vi "Read Scrubber.vi"(8 "error in":errorcluster, 11 "Options in":refnum<class "Options.lvclass">) -> (0 "error out":errorcluster, 2 "Scrubber":refnum<class "Scrubber.lvclass">, 3 "Options out":refnum<class "Options.lvclass">)   [LabVIEW 2020, in "Approval Tests.lvlib" / "Options.lvclass"]
uses:
  Options.lvclass
  Scrubber/Scrubber.lvclass
  Options.lvclass/Options.ctl
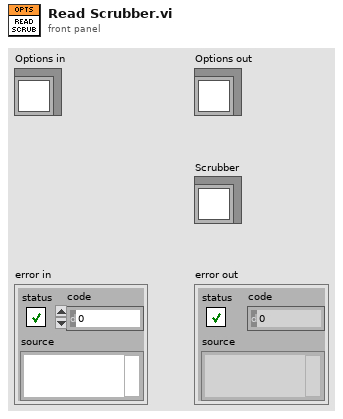
[diagram p1: front panel]
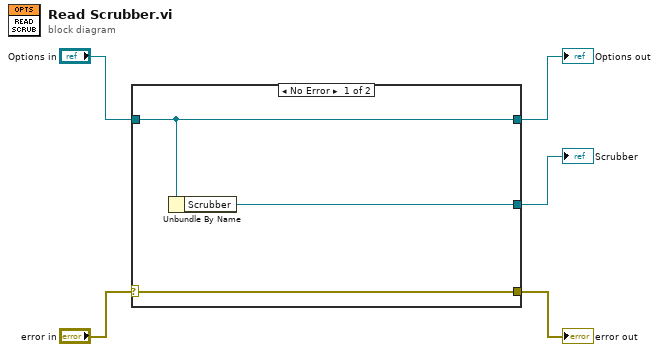
[diagram p0: block diagram]
diagram:
  n1 = case shown="No Error" "error in" {
    selector: "error in" -> [w8 w10]
    tunnel: [w8 w10] -> w4
    tunnel: [w7 w9] -> w2
    tunnel: "Options in" -> [w7 w9]
    tunnel: [w6 _] -> w1
    frame No Error {
      n2 = Unbundle By Name(w7) -> ("Scrubber"=w6:refnum<class "Scrubber.lvclass">)
    }
    frame Error {
    }
  }
  "error out" <- w4
  "Options out" <- w2
  "Scrubber" <- w1
